vi "SpectrumGraph2.vi"() -> ()   [LabVIEW 2014]
uses:
  <vilib>/Utility/file.llb/Write To Spreadsheet File (DBL).vi
  <vilib>/Utility/file.llb/Read From Spreadsheet File (DBL).vi
panel:
  in  "Divider Factor":i32=20
  out "Power (W)":dbl[](array[numeric])=[0.001849, 0.000486, 0.00147, 0.000911, 0.000426, 0.001457, 0.001637, 0.000812, 0.00051, 0.000869, 0.000693, 0.001267, 0.001408, 0.002795, 0.001834, 0.001779, 0.003232, 0.002663, 0.003553, 0.003418, 0.003261, 0.003564, 0.0039, 0.004526, 0.004925, 0.005661, 0.005805, 0.006052, 0.006167, 0.007025, 0.007025, 0.007542, 0.007525, 0.008179, 0.008619, 0.009403, 0.009665, 0.010586, 0.012676, 0.012357, 0.012529, 0.013535, 0.014379, 0.014735, 0.015779, 0.016625, 0.017686, 0.01719, 0.018394, 0.018698, 0.019464, 0.019467, 0.020764, 0.021079, 0.021148, 0.021827, 0.022892, 0.023342, 0.024, 0.024178, 0.025309, 0.024739, 0.026684, 0.026911, 0.027151, 0.027802, 0.029099, 0.029007, 0.028884, 0.030017, 0.030234, 0.030422, 0.03135, 0.031456, 0.032752, 0.032857, 0.033197, 0.03376, 0.034069, 0.034306, 0.035273, 0.035229, 0.035974, 0.03659, 0.036046, 0.035688, 0.037667, 0.037535, 0.037488, 0.038741, 0.038455, 0.038197, 0.03923, 0.041409, 0.040494, 0.041576, 0.041096, 0.041314, 0.040674, 0.03998, 0.040794, 0.041023, 0.040902] format="%#_6f"
  out "Pulse Energy (J)":dbl[](array[numeric])=[9.245e-05, 2.43e-05, 7.35e-05, 4.555e-05, 2.13e-05, 7.285e-05, 8.185e-05, 4.06e-05, 2.5500000000000003e-05, 4.345e-05, 3.465e-05, 6.335e-05, 7.04e-05, 0.00013975, 9.169999999999999e-05, 8.895e-05, 0.0001616, 0.00013315, 0.00017765, 0.0001709, 0.00016305, 0.0001782, 0.000195, 0.00022629999999999997, 0.00024625, 0.00028305, 0.00029025000000000003, 0.0003026, 0.00030835, 0.00035125, 0.00035125, 0.0003771, 0.00037624999999999996, 0.00040895000000000005, 0.00043095, 0.00047015, 0.00048325, 0.0005293, 0.0006338, 0.00061785, 0.00062645, 0.00067675, 0.00071895, 0.00073675, 0.0007889500000000001, 0.0008312500000000001, 0.0008843, 0.0008595, 0.0009197000000000001, 0.0009349, 0.0009731999999999999, 0.0009733500000000001, 0.0010382, 0.0010539500000000001, 0.0010574, 0.00109135, 0.0011446, 0.0011671000000000001, 0.0012000000000000001, 0.0012089000000000002, 0.00126545, 0.0012369500000000001, 0.0013342, 0.00134555, 0.0013575500000000001, 0.0013901, 0.00145495, 0.00145035, 0.0014442, 0.00150085, 0.0015117, 0.0015211, 0.0015675, 0.0015727999999999998, 0.0016376000000000001, 0.00164285, 0.0016598499999999998, 0.0016879999999999998, 0.00170345, 0.0017153000000000001, 0.0017636499999999999, 0.0017614500000000001, 0.0017986999999999999, 0.0018295, 0.0018023000000000002, 0.0017843999999999998, 0.00188335, 0.00187675, 0.0018744, 0.0019370499999999998, 0.0019227500000000002, 0.00190985, 0.0019615, 0.00207045, 0.0020247, 0.0020788, 0.0020548, 0.0020656999999999997, 0.0020337000000000003, 0.001999, 0.0020396999999999998, 0.00205115, 0.0020451]
  out "Total Specs":i32=103
  in  "Load Spectrum":bool
  out "Spectrun File out":string="Andre-3C12D-SpecGraphs Feb-13-2021 Time 22-28.spg"
  out "Especs reduced":i32=10
  in  "Select Spectrum Graph":dbl(slide) step=1.0 scale=0.0..100.0
  out "Waveform Graph":dbl[][](graph)
  out "Points reduced":i32=2048
  out "Points":i32=2048
  in  "Reduce Array Size (2^nTimes)":i32
  out "XY Graph":cluster{dbl[], dbl[]}(graph)
  out "Spectrun File in":string="Andre-3C12D-Spectrum Data out-10-2020 Time 04-11.spt"
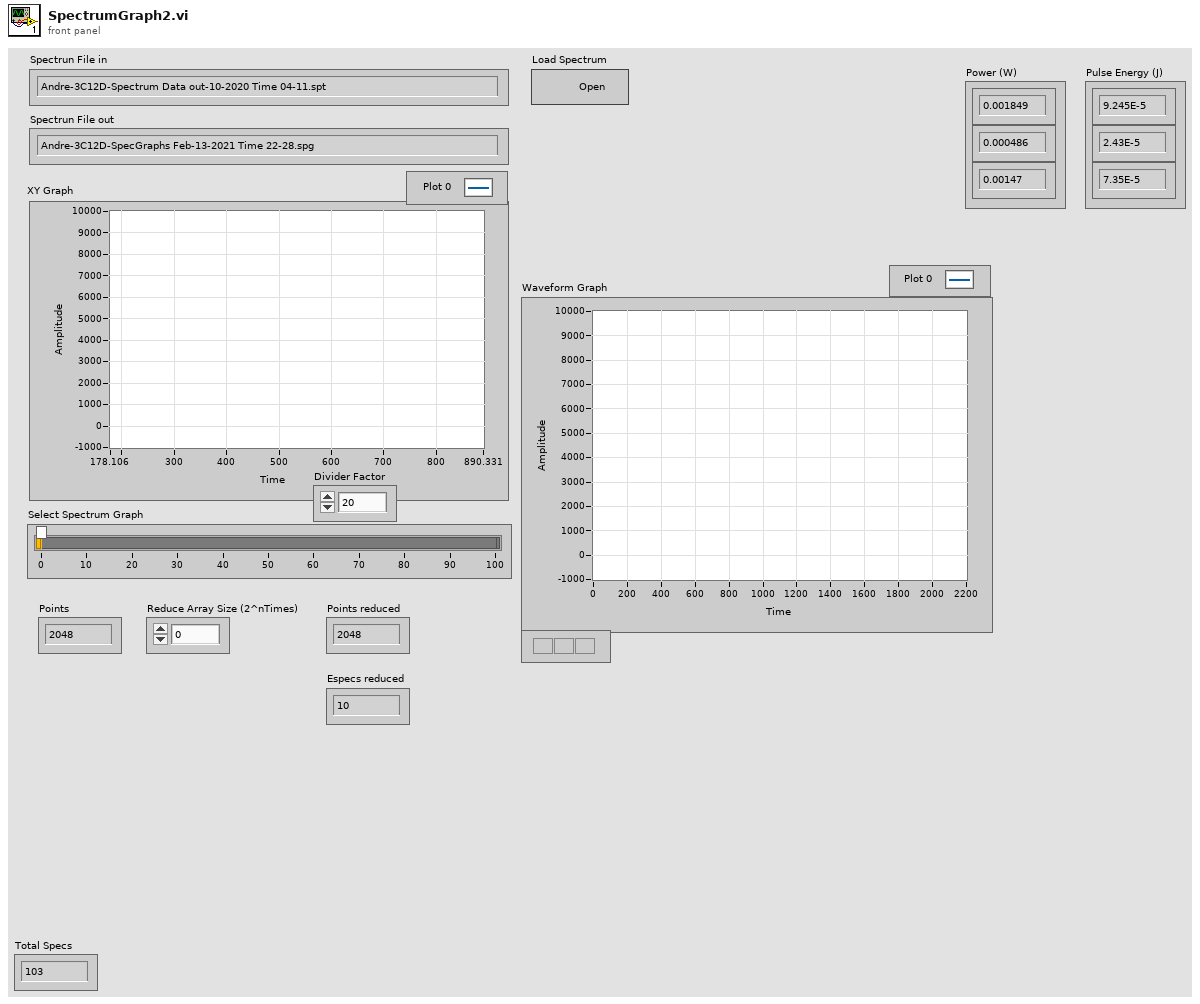
[diagram p1: front panel]
types:
  T1 = enum16{"waitForEvent", "loadFile", "reduceSpecs", "reducePoints", "saveFile"}
  T2 = enum16{"open", "replace", "create", "open or create", "replace or create", "replace or create with confirmation"}
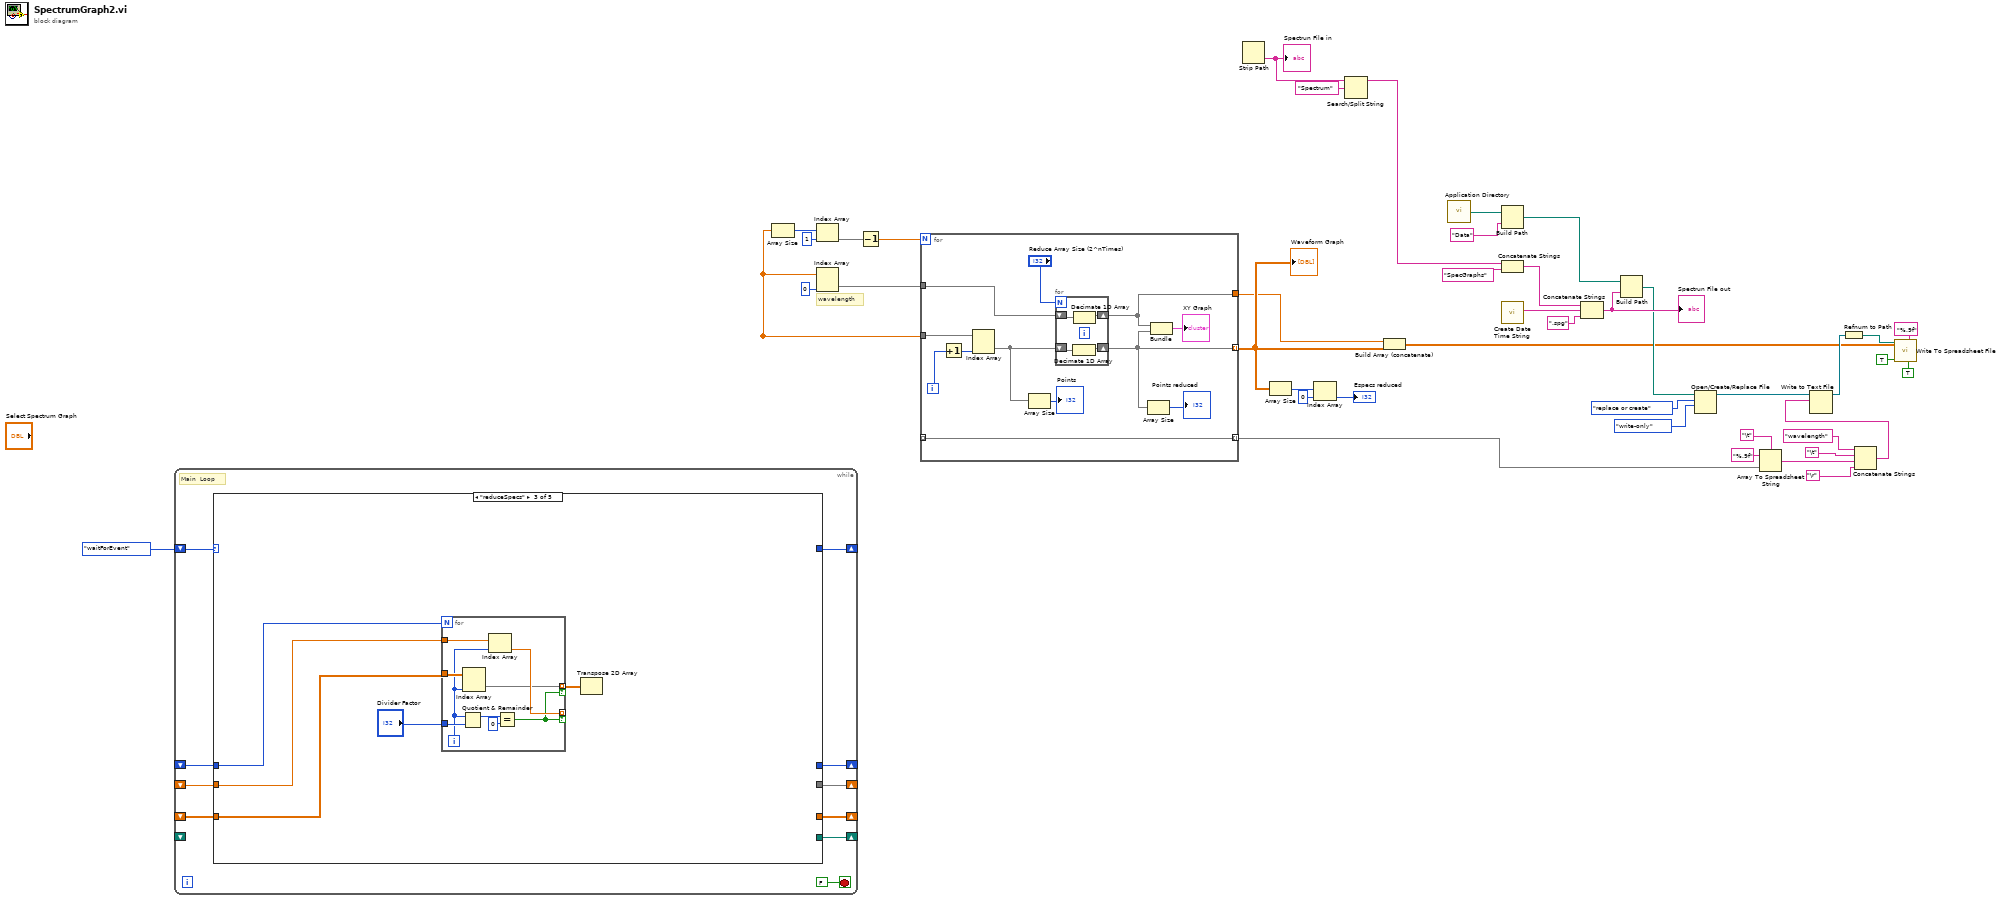
[diagram p0: block diagram]
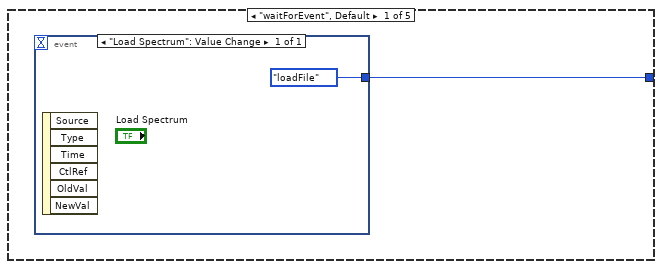
[diagram p2: hidden frame]
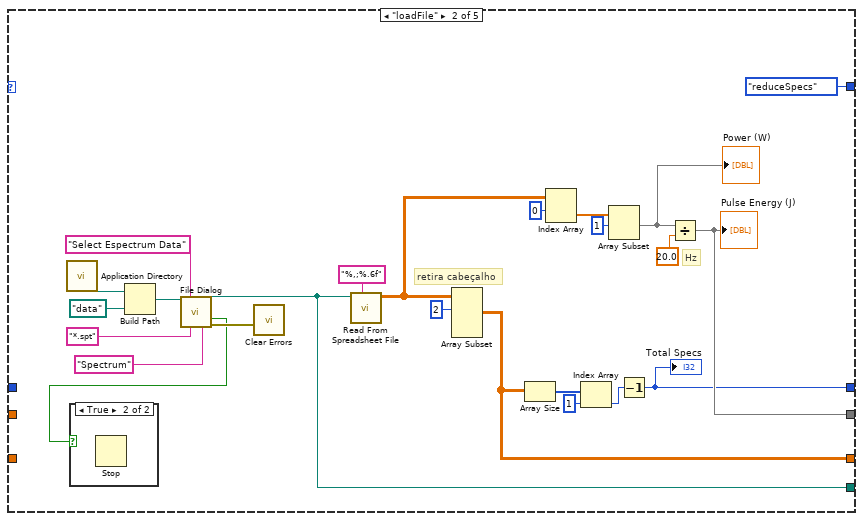
[diagram p3: hidden frame]
diagram:
  # "wavelength"
  n1 = while {
    shift-right: [w52] -> _
    shift-left: T1."waitForEvent" -> [w53]
    shift-right: [w51] -> _
    shift-left: _ -> [w50]
    shift-right: [w49] -> _
    shift-left: _ -> [w48]
    shift-right: [w47] -> _
    shift-left: _ -> [_]
    shift-right: [w46] -> _
    shift-left: _ -> [w45]
    stop <- FALSE stop-if-true
    # "Main  Loop"
    n2 = case shown="\"reduceSpecs\"" w53 {
      tunnel: [w55 T1."reduceSpecs" _ _ _] -> w52
      tunnel: [_ w60 _ _ _] -> w49
      tunnel: [_ w59 _ _ _] -> w46
      tunnel: [_ w58 _ _ _] -> w51
      tunnel: [_ w57 _ _ _] -> w47
      tunnel: w50 -> [_ _ w83 _ _]
      tunnel: w48 -> [_ _ w82 _ _]
      tunnel: w45 -> [_ _ w81 _ _]
      frame "waitForEvent", Default {
        n3 = event shown="[0] \"Load Spectrum\": Value Change" {
          selector: _ -> [_]
          dyn-events: _ -> [_]
          timeout: _ -> [_]
          tunnel: [T1."loadFile"] -> w55
          event "Load Spectrum": Value Change {
            n4 = event-data() -> ()  [unwired: 1 in, 6 out]
          }
        }
      }
      frame "loadFile" {
        # "Hz"
        # "retira cabeçalho"
        n5 = call <vilib>:"Application Directory.vi"() -> ("Application Directory"=w75:path)
        n6 = Build Path(base path=w75, name or relative path=path "data") -> (appended path=w74:path)
        n7 = call "File Dialog"("start path"=w74, "prompt"="Select Espectrum Data", "pattern (all files)"="*.spt", "pattern label"="Spectrum") -> ("selected path"=w57:path, "cancelled"=w72:bool, "error out"=w73:errorcluster)  [unwired: 8 in, 1 out]
        n8 = case shown="True" w72 {
          frame False {
          }
          frame True {
            n9 = Stop() -> ()  [unwired: 1 in]
          }
        }
        n10 = call <vilib>:"Clear Errors.vi"("error in (no error)"=w73) -> ()  [unwired: 5 in, 2 out]
        n11 = call-poly <vilib>:"Read From Spreadsheet File.vi"("format (%.3f)"="%,;%.6f", "file path (dialog if empty)"=w57) -> ("all rows"=w69:dbl[][])  [unwired: 5 in, 4 out]
        n12 = Array Subset(array=w69, index (row)=2 ("index")) -> (w58:dbl[][])  [unwired: 3 in]
        n13 = Array Size(array=w58) -> (size(s)=w63:i32[])
        n14 = Index Array(array=w69, index (row)=0) -> (element=w67:dbl[])  [unwired: 1 in]
        n15 = Index Array(array=w63, index=1) -> (element=w61:i32)
        n16 = Array Subset(array=w67, index=1) -> (w64:dbl[])  [unwired: 1 in]
        "Power (W)" <- w64
        n17 = Decrement(x=w61) -> (x-1=w59:i32)
        "Total Specs" <- w59
        n18 = Divide(x=w64, y=20.0) -> (x/y=w60:dbl[])
        "Pulse Energy (J)" <- w60
      }
      frame "reduceSpecs" {
        n19 = for {
          N: w81 -> [_]
          tunnel: w83 -> [w92]
          tunnel: "Divider Factor" -> [w95]
          tunnel: w82 -> [w91]
          tunnel: [w89] -> _ mode=indexing if=w87
          tunnel: [w88] -> w85 mode=indexing if=w87
          i -> [w90]
          n20 = Quotient & Remainder(x=w90, y=w95) -> (x-y*floor(x/y)=w94:i32)  [unwired: 1 out]
          n21 = Index Array(array=w92, index (col)=w90) -> (element=w88:dbl[])  [unwired: 1 in]
          n22 = Index Array(array=w91, index=w90) -> (element=w89:dbl)
          n23 = Equal?(x=w94, y=0) -> (x = y?=w87:bool)
        }
        n24 = Transpose 2D Array(2D array=w85) -> (transposed array=w84:dbl[][])
      }
      frame "reducePoints" {
      }
      frame "saveFile" {
      }
    }
  }
  n25 = Array Size() -> (array=w2:dbl[], size(s)=w43:i32)
  n26 = Index Array(array=w43, index=1) -> (element=w38)
  n27 = Index Array(array=w2, index (col)=0 ("disabled index (col)")) -> (element=w40)  [unwired: 1 in]
  n28 = Decrement(x=w38) -> (x-1=w37:dbl)
  n29 = for {
    N: w37 -> [_]
    tunnel: w2 -> [w107]
    tunnel: w40 -> [w103]
    tunnel: [w99] -> w6
    tunnel: [w98] -> w8 mode=indexing
    tunnel: [w96] -> w5 mode=indexing
    tunnel: [w96] -> w7 mode=indexing
    i -> [w97]
    n30 = Increment(x=w97) -> (x+1=w106:i32)
    n31 = Index Array(array=w107, index (col)=w106) -> (element=w102)  [unwired: 1 in]
    n32 = Array Size(array=w102) -> (size(s)=→"Points":i32)
    n33 = for {
      N: "Reduce Array Size (2^nTimes)" -> [_]
      shift-right: [w109] -> w99
      shift-left: w103 -> [w111]
      shift-right: [w108] -> w98
      shift-left: w102 -> [w110]
      n34 = Decimate 1D Array(w110) -> (w108:dbl[])  [unwired: 1 out]
      n35 = Decimate 1D Array(w111) -> (w109:dbl[])  [unwired: 1 out]
    }
    n36 = Array Size(array=w98) -> (size(s)=→"Points reduced":i32)
    n37 = Bundle(w99, w98) -> (→"XY Graph":cluster{dbl[], dbl[]})  [unwired: 1 in]
  }
  "Waveform Graph" <- w8
  n38 = Strip Path() -> (path=w41:path, name=w36:string)  [unwired: 1 out]
  "Spectrun File in" <- w36
  n39 = Array Size(array=w8) -> (size(s)=w39:i32[])
  n40 = Index Array(array=w39, index=0) -> (element=→"Especs reduced":i32)
  n41 = Search/Split String(string=w36, search string/char (-)="Spectrum") -> (substring before match=w26:string)  [unwired: 1 in, 2 out]
  n42 = Build Array (concatenate)(w6, w8) -> (w9:dbl[][])
  n43 = call <vilib>:"Application Directory.vi"() -> ("Application Directory"=w28:path)
  n44 = Build Path(base path=w28, name or relative path="Data" ("prompt (Create Folder)")) -> (appended path=w27:path)
  n45 = Concatenate Strings(w26, "SpecGraphs" ("string")) -> (w30:string)
  n46 = call "Create Date Time String.vi"() -> ("Date/Time String"=w34:string)  [unwired: 10 in, 1 out]
  n47 = Concatenate Strings(w30, w34, ".spg" ("string")) -> (w32:string)
  "Spectrun File out" <- w32
  n48 = Build Path(base path=w27, name or relative path=w32) -> (appended path=w11:path)
  n49 = Open/Create/Replace File(file path (use dialog)=w11, operation (0:open)=T2."replace or create", access (0:read/write)=enum16{"read/write", "read-only", "write-only"}."write-only") -> (refnum out=w21:refnum<file>)  [unwired: 3 in, 2 out]
  n50 = Array To Spreadsheet String(delimiter (Tab)="\t", array=w7, 3:"%.9f" ("format string")) -> (spreadsheet string=w16:string)
  n51 = Concatenate Strings("wavelength" ("string"), "\t", w16, "\r") -> (w15:string)
  n52 = Write to Text File(file (use dialog)=w21, text=w15) -> (refnum out=w20:refnum<file>)  [unwired: 2 in, 2 out]
  n53 = Refnum to Path(1:w20) -> (0:w25:path)
  n54 = call-poly <vilib>:"Write To Spreadsheet File.vi"("transpose? (no:F)"=TRUE, "format (%.3f)"="%.9f" ("format string"), "append to file? (new file:F)"=TRUE, "2D data"=w9, "file path (dialog if empty)"=w25) -> ()  [unwired: 3 in, 1 out]
